vi "Get_Mean_A+P.vi"(5 "Wait [s]":dbl, 6 "Frequency [Hz]":dbl, 7 "error in (no error)":errorcluster) -> (0 "Mean Amplitude":dbl, 1 "Error Amplitude":dbl, 2 "Mean Phase Shift":dbl, 3 "error out":errorcluster, 4 "Error Phase Shift":dbl)   [LabVIEW 2010]
uses:
  <vilib>/Analysis/NI_AALBase.lvlib
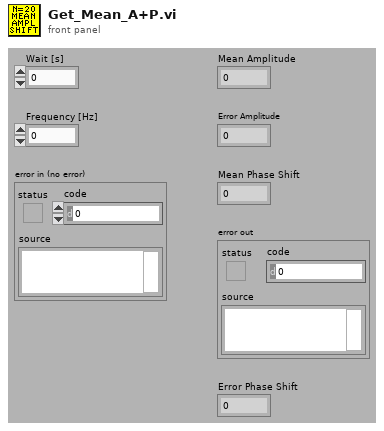
[diagram p1: front panel]
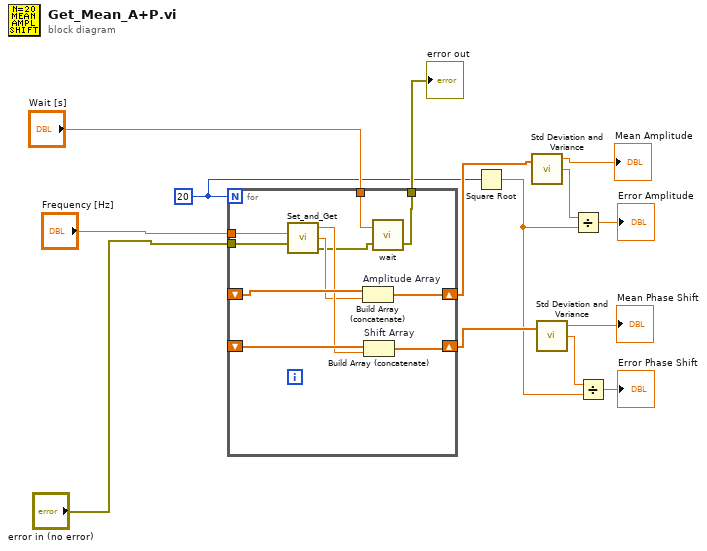
[diagram p0: block diagram]
diagram:
  w1 = 20
  n1 = for {
    N: w1 -> [_]
    tunnel: "Frequency [Hz]" -> [w25]
    tunnel: "error in (no error)" -> [w24]
    shift-right: [w20] -> w4
    shift-left: _ -> [w21]
    shift-right: [w23] -> w11
    shift-left: _ -> [w22]
    tunnel: [w16] -> w2
    tunnel: "Wait [s]" -> [w15]
    n2 = call "Set_and_Get.vi"("error in (no error)"=w24, "Frequency"=w25) -> ("error out"=w17:errorcluster, "Amplitude"=w18:dbl, "Phase Shift"=w19:dbl)
    n3 = Build Array (concatenate) "Amplitude Array"(w22, w18) -> (w23:dbl[])
    n4 = Build Array (concatenate) "Shift Array"(w21, w19) -> (w20:dbl[])
    n5 = call "wait.vi"("error in"=w17, "Wartezeit in Sek"=w15) -> ("error out"=w16:errorcluster)  [unwired: 1 in]
  }
  "error out" <- w2
  n6 = Square Root(x=w1) -> (sqrt(x)=w3:dbl)
  n7 = call <vilib>:"Std Deviation and Variance.vi"("X"=w11) -> ("mean"=→"Mean Amplitude":dbl, "standard deviation"=w8:dbl)  [unwired: 1 in, 1 out]
  n8 = call <vilib>:"Std Deviation and Variance.vi"("X"=w4) -> ("mean"=→"Mean Phase Shift":dbl, "standard deviation"=w7:dbl)  [unwired: 1 in, 1 out]
  n9 = Divide(x=w8, y=w3) -> (x/y=→"Error Amplitude":dbl)
  n10 = Divide(x=w7, y=w3) -> (x/y=→"Error Phase Shift":dbl)
